vi "playVlc.vi"(8 "error in (no error)":errorcluster, 10 "playVlc":string, 11 "VlcPlayer in":refnum<class "VlcPlayer.lvclass">) -> (0 "error out":errorcluster, 3 "VlcPlayer out":refnum<class "VlcPlayer.lvclass">)   [LabVIEW 2018, in "VlcPlayer.lvclass"]
uses:
  VlcPlayer.lvclass
  ConsoleOut/Print Options.ctl
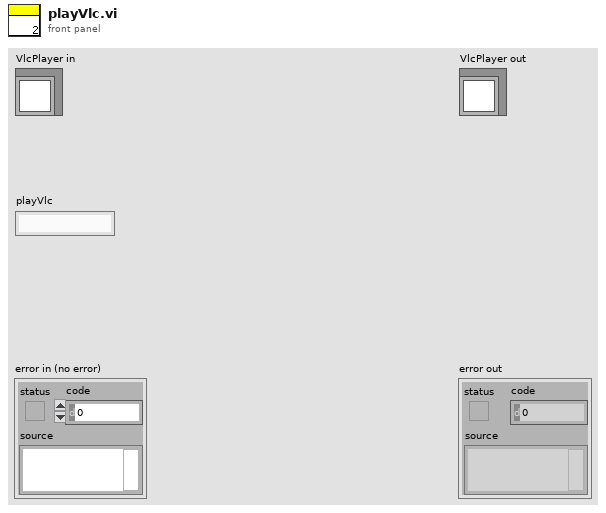
[diagram p1: front panel]
types:
  T1 = typedef "Print Options.ctl" = enum16{"Create", "Get Reference", "Print", "Print Header", "Close"}
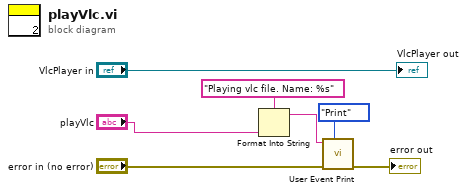
[diagram p0: block diagram]
diagram:
  n1 = Format Into String(format string="Playing vlc file. Name: %s", "playVlc") -> (resulting string=w2:string)  [unwired: 2 in, 1 out]
  n2 = call "User Event Print.vi"("Options"=Print_Options."Print", "error in (no error)"="error in (no error)", "String to Print"=w2) -> ("error out"=→"error out":errorcluster)  [unwired: 7 in, 1 out]
  "VlcPlayer out" <- "VlcPlayer in"
